vi "Configure Alternation Trigger Characteristics.vi"(0 "VISA resource name":refnum<visa-resource-name>, 1 "Trigger Level (0.0 V)":dbl, 2 "Sensitivity (0.1 V)":dbl=0.1, 3 "Enable High Frequency Filter (F: Disable)":bool, 5 "Source Channel (0: Source A)":u16(ring) items=["Source A", "Source B"], 7 "Trigger Coupling (0: DC)":u16(ring) items=["DC", "AC", "Low Frequency Reject"], 9 "Trigger Holdoff (1E-7 s)":dbl=1e-07, 11 "error in (no error)":errorcluster, 12 "Time per Division (1E-6 s)":dbl=1e-06, 13 "Time Delay (0.0 s)":dbl) -> (4 "VISA resource name out":refnum<visa-resource-name>, 15 "error out":errorcluster)   [LabVIEW 2010, in "Agilent DSO1000 Series.lvlib"]
doc: "Configures alternation trigger settings. Specifies the trigger type and general setting on specified channel."
uses:
  <instrlib>/Agilent DSO1000 Series/Agilent DSO1000 Series.lvlib
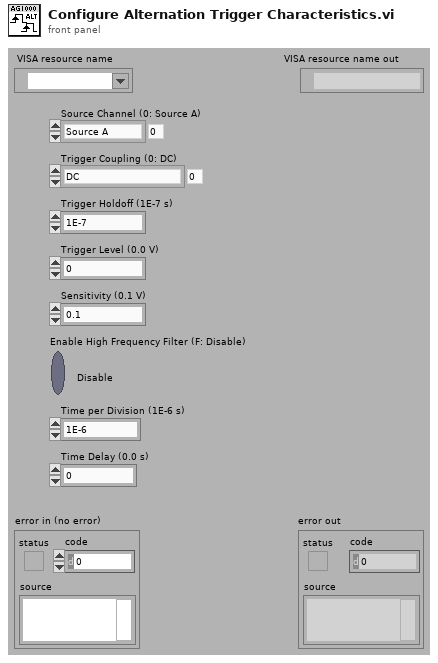
[diagram p1: front panel]
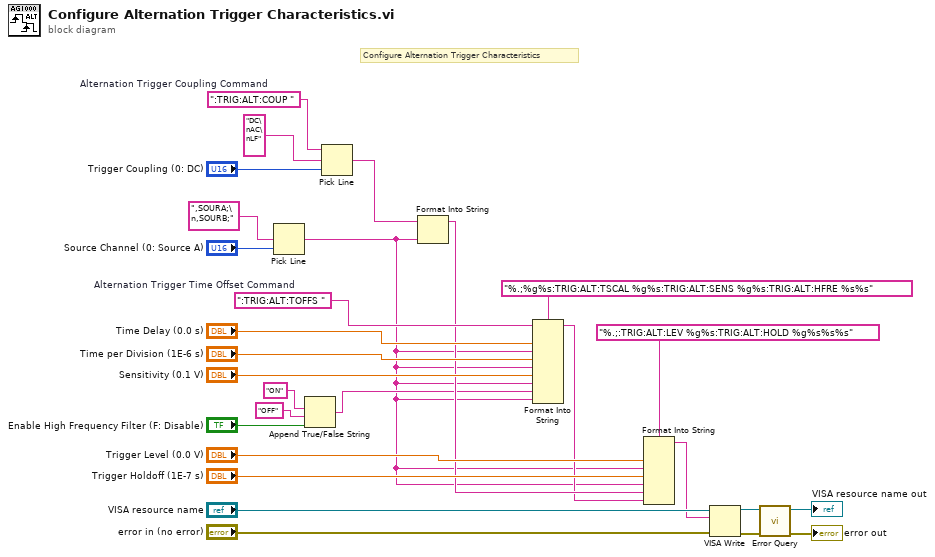
[diagram p0: block diagram]
diagram:
  w17 = ":TRIG:ALT:TOFFS "  # Alternation Trigger Time Offset Command
  w21 = ":TRIG:ALT:COUP "  # Alternation Trigger Coupling Command
  # "Configure Alternation Trigger Characteristics"
  n1 = Pick Line(multi-line string=",SOURA;\n,SOURB;", line index="Source Channel (0: Source A)") -> (output string=w1:string)  [unwired: 1 in]
  n2 = Append True/False String(1:"Enable High Frequency Filter (F: Disable)", 2:"OFF" ("false string"), 3:"ON" ("true string")) -> (0:w2:string)  [unwired: 1 in]
  n3 = Pick Line(string ("")=w21, multi-line string="DC\nAC\nLF", line index="Trigger Coupling (0: DC)") -> (output string=w22:string)
  n4 = Format Into String(initial string=w22, w1) -> (resulting string=w8:string)  [unwired: 2 in, 1 out]
  n5 = Format Into String(format string="%.;%g%s:TRIG:ALT:TSCAL %g%s:TRIG:ALT:SENS %g%s:TRIG:ALT:HFRE %s%s", initial string=w17, "Time Delay (0.0 s)", w1, "Time per Division (1E-6 s)", w1, "Sensitivity (0.1 V)", w1, w2, w1) -> (resulting string=w7:string)  [unwired: 1 in, 1 out]
  n6 = Format Into String(format string="%.;:TRIG:ALT:LEV %g%s:TRIG:ALT:HOLD %g%s%s%s", "Trigger Level (0.0 V)", w1, "Trigger Holdoff (1E-7 s)", w1, w8, w7) -> (resulting string=w6:string)  [unwired: 2 in, 1 out]
  n7 = VISA Write(VISA resource name="VISA resource name", write buffer=w6, error in (no error)="error in (no error)") -> (VISA resource name out=w20:refnum<visa-resource-name>, error out=w19:errorcluster)  [unwired: 1 out]
  n8 = call <instrlib>:"Error Query.vi"("error in (no error)"=w19, "VISA resource name"=w20) -> ("error out"=→"error out":errorcluster, "VISA resource name out"=→"VISA resource name out":refnum<visa-resource-name>)  [unwired: 6 in, 2 out]
